vi "AutoSequencer.vi"(0 "Auto Test Heading In (deg)":dbl, 1 "Mobility Advance In":bool, 2 "Mobility Step In":i32, 3 "Subsystem Timer In (ms)":u32, 4 "Subsystem Advance In":bool, 5 "Subsystem Step In":i32, 6 "Auto Error In":errorcluster, 8 "Reinit Sequencer":bool) -> (12 "Auto Error Out":errorcluster, 14 "Auto Test Heading Out (deg)":dbl, 15 "Mobility Advance Out":bool, 16 "Mobility Step Out":i32, 17 "Subsystem Timer Out (ms)":u32, 18 "Subsystem Advance Out":bool, 19 "Subsystem Step Out":i32)   [LabVIEW 2019]
uses:
  dda54508-1252-4ecd-8301-0edc88a214cb.vi
  36410131-339f-4f96-8020-6b3055e7e82c.vi
  constants.vi
  dsdata.vi
  sensors.vi
  autoninfo.vi
  <vilib>/Rock Robotics/Network Tables/NT Write String.vi
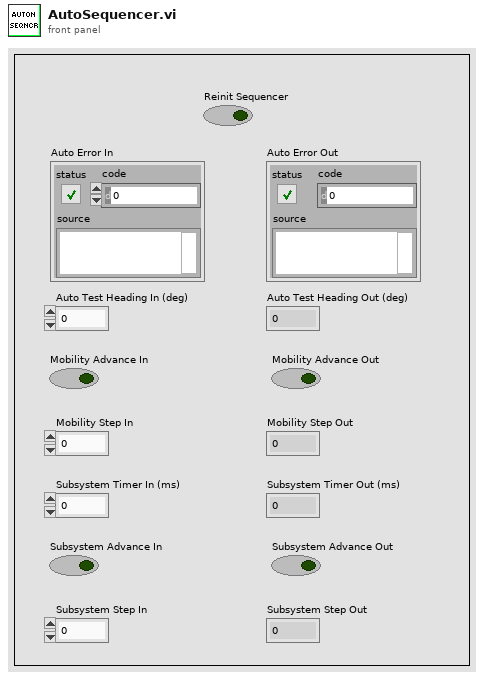
[diagram p1: front panel]
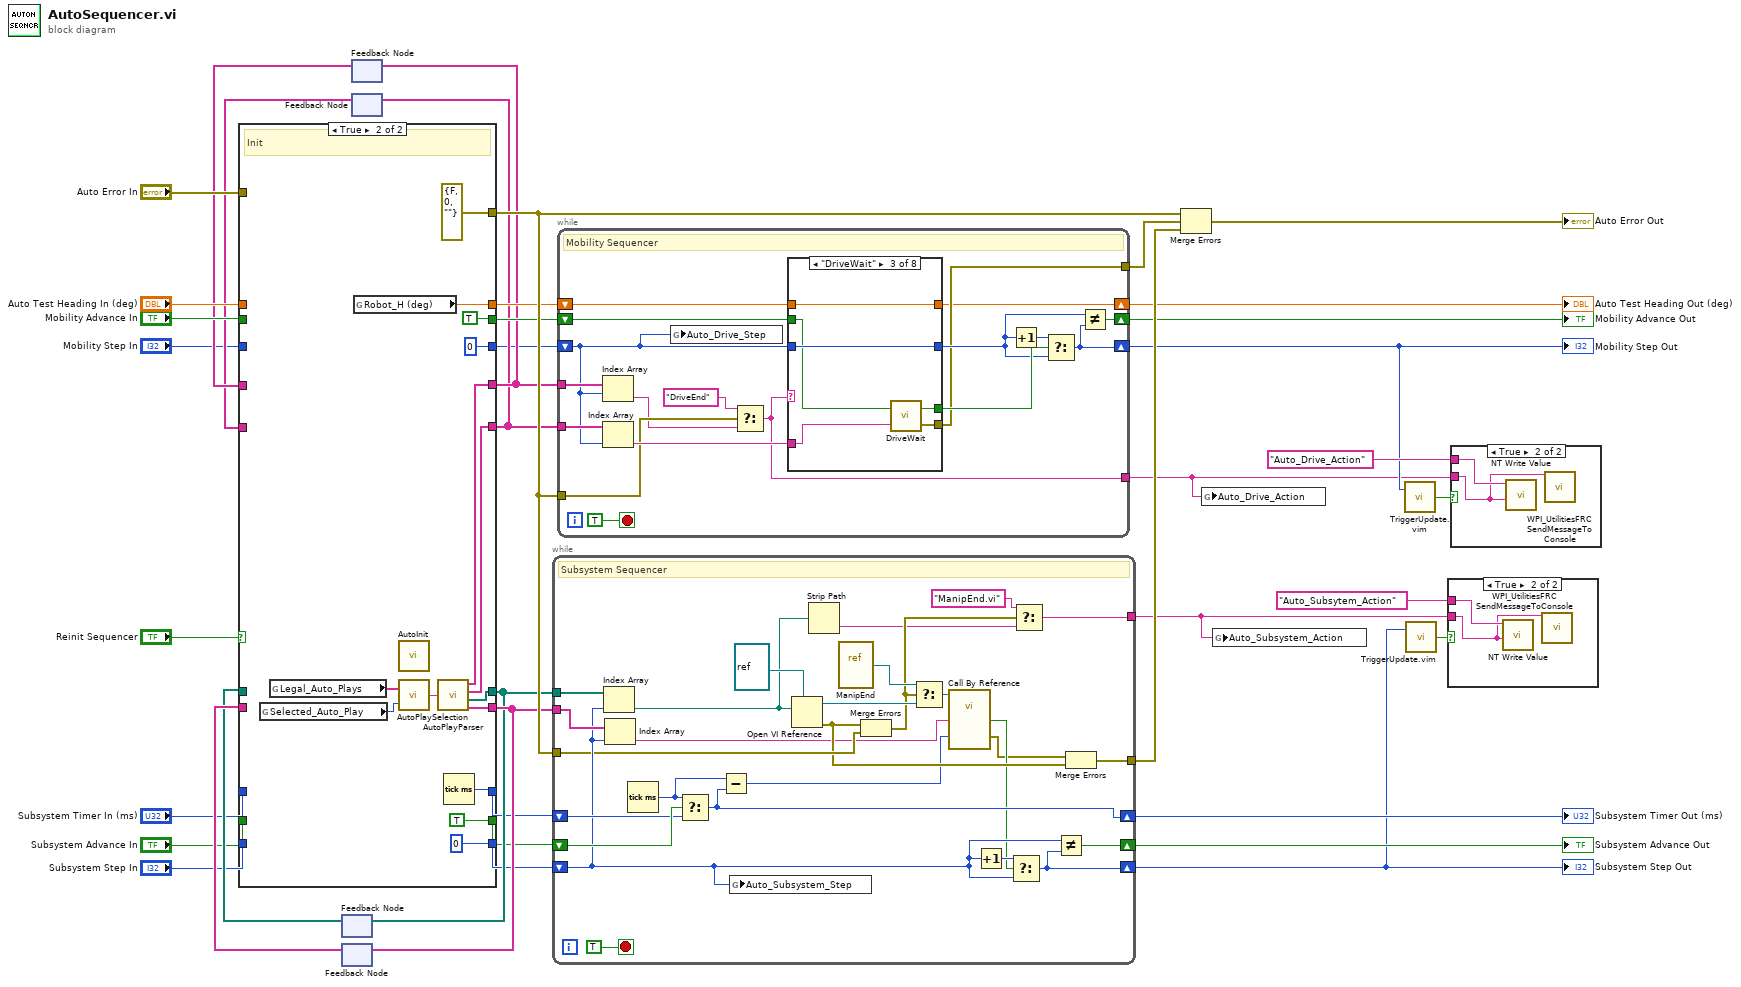
[diagram p0: block diagram]
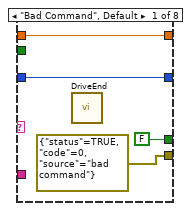
[diagram p4: hidden frame]
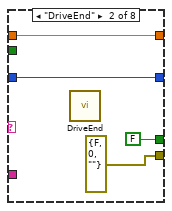
[diagram p5: hidden frame]
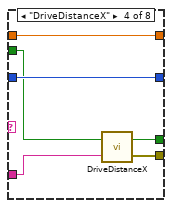
[diagram p6: hidden frame]
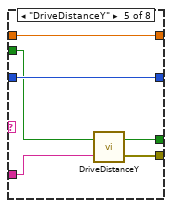
[diagram p7: hidden frame]
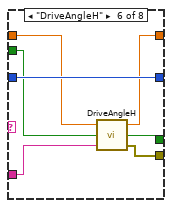
[diagram p8: hidden frame]
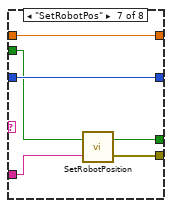
[diagram p9: hidden frame]
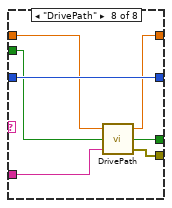
[diagram p10: hidden frame]
diagram:
  n1 = feedback #1() -> (w16:path[])  [unwired: 1 in]
  n2 = feedback #2() -> (w17:string[])  [unwired: 1 in]
  n3 = feedback #3() -> (w23:string[])  [unwired: 1 in]
  n4 = feedback #4() -> (w22:string[])  [unwired: 1 in]
  n5 = case shown="True" "Reinit Sequencer" {
    tunnel: "Subsystem Step In" -> [w47 _]
    tunnel: "Subsystem Advance In" -> [w48 _]
    tunnel: "Subsystem Timer In (ms)" -> [w49 _]
    tunnel: [w49 w63] -> w8
    tunnel: [w48 TRUE ("Advance Trigger")] -> w11
    tunnel: [w47 0] -> w12
    tunnel: [w46 w56] -> w14
    tunnel: [w45 w60] -> w15
    tunnel: w16 -> [w46 _]
    tunnel: w17 -> [w45 _]
    tunnel: [w44 0] -> w18
    tunnel: "Mobility Step In" -> [w44 _]
    tunnel: [w43 w58] -> w20
    tunnel: [w42 w57] -> w21
    tunnel: w22 -> [w43 _]
    tunnel: w23 -> [w42 _]
    tunnel: [w41 TRUE] -> w24
    tunnel: "Mobility Advance In" -> [w41 _]
    tunnel: [w40 w51] -> w31
    tunnel: "Auto Test Heading In (deg)" -> [w40 _]
    tunnel: [w39 errorcluster {"status"=FALSE, "code"=0, "source"=""} ("error constant")] -> w37
    tunnel: "Auto Error In" -> [w39 _]
    frame False {
      # "Pass"
    }
    frame True {
      # "Init"
      n6 = global read "dsdata.vi" "Selected_Auto_Play"() -> (w54:u16)
      n7 = global read "constants.vi" "Legal_Auto_Plays"() -> (w53:string[])
      n8 = global read "sensors.vi" "Robot_H (deg)"() -> (w51:dbl)
      n9 = call "AutoInit.vi"() -> ()  [unwired: 1 in]
      n10 = call "AutoPlaySelection.vi"("Selected Auto Play"=w54, "Auto Plays"=w53) -> ("Autonomous Commands"=w52:string)
      n11 = call "AutoPlayParser.vi"("Auto Play"=w52) -> ("Drive Mode Strings"=w57:string[], "Drive Command Strings"=w58:string[], "Subsystem VI References"=w56:path[], "Subsystem Command Strings"=w60:string[])
      n12 = Tick Count (ms)() -> (millisecond timer value=w63:u32)
    }
  }
  n13 = feedback-in #1(w14) -> ()
  n14 = feedback-in #2(w15) -> ()
  n15 = feedback-in #3(w21) -> ()
  n16 = feedback-in #4(w20) -> ()
  n17 = while {
    tunnel: w14 -> [w82]
    shift-right: [w88] -> w3
    shift-left: w12 -> [w77]
    shift-right: [w87] -> w6
    shift-left: w11 -> [w86]
    shift-right: [w84] -> w5
    shift-left: w8 -> [w85]
    tunnel: w15 -> [w81]
    tunnel: [w64] -> w1
    tunnel: [w78] -> w38
    tunnel: w37 -> [w76]
    stop <- TRUE stop-if-true
    # "Subsystem Sequencer"
    n18 = Index Array(array=w82, index=w77) -> (element=w69:path)
    n19 = Index Array(array=w81, index=w77) -> (element=w73:string)
    n20 = Tick Count (ms)() -> (millisecond timer value=w83:u32)
    n21 = Select(t=w83, s=w86, f=w85) -> (s? t:f=w84:u32)
    n22 = Subtract(x=w83, y=w84) -> (x-y=w72:u32)
    n23 = global write "autoninfo.vi" "Auto_Subsystem_Step"(w77) -> ()
    n24 = Open VI Reference(type specifier VI Refnum (for type only)=refnum<vi> refnum, vi path=w69) -> (vi reference=w80:refnum<vi>, error out=w75:errorcluster)  [unwired: 4 in]
    n25 = Strip Path(path=w69) -> (name=w65:string)  [unwired: 1 out]
    n26 = vi-ref "ManipEnd.vi"() -> (w79:refnum<vi>)
    n27 = Merge Errors(w75, w76) -> (w67:errorcluster)
    n28 = Select(t=w79, s=w67, f=w80) -> (s? t:f=w68:refnum<vi>)
    n29 = call-by-ref "?"(reference=w68, "Time Since Latch"=w72, "Instruction String"=w73) -> ("Error Out"=w70:errorcluster, "Advance Trigger"=w71:bool)  [unwired: 1 in, 2 out]
    n30 = Increment(x=w77) -> (x+1=w90:i32)
    n31 = Select(t=w90, s=w71, f=w77) -> (s? t:f=w88:i32)
    n32 = Select(t="ManipEnd.vi", s=w67, f=w65) -> (s? t:f=w64:string)
    n33 = Not Equal?(x=w77, y=w88) -> (x != y?=w87:bool)
    n34 = Merge Errors(w70, w75) -> (w78:errorcluster)
  }
  "Subsystem Step Out" <- w3
  "Subsystem Advance Out" <- w6
  "Subsystem Timer Out (ms)" <- w5
  n35 = while {
    shift-right: [w103] -> w4
    shift-left: w18 -> [w95]
    tunnel: w21 -> [w106]
    tunnel: w20 -> [w105]
    shift-right: [w102] -> w25
    shift-left: w24 -> [w101]
    tunnel: [w91] -> w2
    shift-right: [w92] -> w33
    shift-left: w31 -> [w93]
    tunnel: w37 -> [w98]
    tunnel: [w94] -> w36
    stop <- TRUE stop-if-true
    # "Mobility Sequencer"
    n36 = Index Array(array=w106, index=w95) -> (element=w97:string)
    n37 = Index Array(array=w105, index=w95) -> (element=w104:string)
    n38 = global write "autoninfo.vi" "Auto_Drive_Step"(w95) -> ()
    n39 = Select(t="DriveEnd", s=w98, f=w97) -> (s? t:f=w91:string)
    n40 = case shown="\"DriveWait\"" w91 {
      tunnel: w95 -> [w112 w116 w122 w128 w134 w141 w147 w154]
      tunnel: [w112 w116 w122 w128 w134 w141 w147 w154] -> w99
      tunnel: w104 -> [_ _ w119 w126 w131 w138 w145 w152]
      tunnel: [FALSE ("Increment") FALSE ("Increment") w121 w125 w133 w140 w146 w150] -> w100
      tunnel: w101 -> [_ _ w120 w127 w132 w139 w144 w153]
      tunnel: [errorcluster {"status"=TRUE, "code"=0, "source"="bad command"} ("Path Follow Error") errorcluster {"status"=FALSE, "code"=0, "source"=""} ("Path Follow Error") w117 w123 w129 w136 w142 w151] -> w94
      tunnel: [w110 w114 w118 w124 w130 w137 w143 w149] -> w92
      tunnel: w93 -> [w110 w114 w118 w124 w130 w135 w143 w148]
      frame "Bad Command", Default {
        n41 = call "DriveEnd.vi"() -> ()  [unwired: 2 in]
      }
      frame "DriveEnd" {
        n42 = call "DriveEnd.vi"() -> ()  [unwired: 2 in]
      }
      frame "DriveWait" {
        n43 = call "DriveWait.vi"("Parameter String"=w119, "Reinit"=w120) -> ("Error Out"=w117:errorcluster, "Increment"=w121:bool)
      }
      frame "DriveDistanceX" {
        n44 = call "DriveDistanceX.vi"("Parameter String"=w126, "Reinit"=w127) -> ("Error Out"=w123:errorcluster, "Increment"=w125:bool)
      }
      frame "DriveDistanceY" {
        n45 = call "DriveDistanceY.vi"("Parameter String"=w131, "Reinit"=w132) -> ("Error Out"=w129:errorcluster, "Increment"=w133:bool)
      }
      frame "DriveAngleH" {
        n46 = call "DriveAngleH.vi"("Parameter String"=w138, "Reinit"=w139, "Auto Test Heading In (deg)"=w135) -> ("Error Out"=w136:errorcluster, "Increment"=w140:bool, "Auto Test Heading Out (deg)"=w137:dbl)
      }
      frame "SetRobotPos" {
        n47 = call "SetRobotPosition.vi"("Parameter String"=w145, "Reinit"=w144) -> ("Error Out"=w142:errorcluster, "Increment"=w146:bool)
      }
      frame "DrivePath" {
        n48 = call "DrivePath.vi"("Parameter String"=w152, "Reinit"=w153, "Auto Test Heading In (deg)"=w148) -> ("Path Follow Error"=w151:errorcluster, "Increment"=w150:bool, "Auto Test Heading Out (deg)"=w149:dbl)
      }
    }
    n49 = Increment(x=w99) -> (x+1=w107:i32)
    n50 = Select(t=w107, s=w100, f=w99) -> (s? t:f=w103:i32)
    n51 = Not Equal?(x=w99, y=w103) -> (x != y?=w102:bool)
  }
  "Auto Test Heading Out (deg)" <- w33
  "Mobility Advance Out" <- w25
  "Mobility Step Out" <- w4
  n52 = Merge Errors(w37, w36, w38) -> (→"Auto Error Out":errorcluster)
  n53 = global write "autoninfo.vi" "Auto_Drive_Action"(w2) -> ()
  n54 = global write "autoninfo.vi" "Auto_Subsystem_Action"(w1) -> ()
  n55 = call "TriggerUpdate.vim"("Trigger"=w4) -> ("Update"=w27:bool)  [unwired: 1 in]
  n56 = call "TriggerUpdate.vim"("Trigger"=w3) -> ("Update"=w29:bool)  [unwired: 1 in]
  n57 = case shown="True" w29 {
    tunnel: w1 -> [_ w155]
    tunnel: "Auto_Subsytem_Action" ("Name") -> [_ w156]
    frame False {
    }
    frame True {
      n58 = call-poly <vilib>:"NT Write Value.vi"("String"=w155, "Name"=w156) -> ()  [unwired: 9 in, 1 out]
      n59 = call <vilib>:"WPI_UtilitiesFRC SendMessageToConsole.vi"("Message"=w155) -> ()  [unwired: 14 in, 1 out]
    }
  }
  n60 = case shown="True" w27 {
    tunnel: w2 -> [_ w157]
    tunnel: "Auto_Drive_Action" ("Name") -> [_ w158]
    frame False {
    }
    frame True {
      n61 = call-poly <vilib>:"NT Write Value.vi"("String"=w157, "Name"=w158) -> ()  [unwired: 9 in, 1 out]
      n62 = call <vilib>:"WPI_UtilitiesFRC SendMessageToConsole.vi"("Message"=w157) -> ()  [unwired: 14 in, 1 out]
    }
  }
